vi "Destroy.vi"(0 "reference in":refnum<class "DP_WebView.lvclass">, 2 "BlankBrowser(True)":bool=TRUE, 5 "Error In":errorcluster) -> (14 "reference out":refnum<class "DP_WebView.lvclass">, 19 "Error Out":errorcluster)   [LabVIEW 2020, in "DP_WebView.lvclass"]
uses:
  DP_WebView.lvclass
  C:/Projects/DependencyViewer/DependencyViewer/DP_WebView_class/data/Microsoft.Web.WebView2.Core.dll
  data/Microsoft.Web.WebView2.Core.dll
  C:/Projects/DependencyViewer/DependencyViewer/DP_WebView_class/data/Microsoft.Web.WebView2.WinForms.dll
  data/Microsoft.Web.WebView2.WinForms.dll
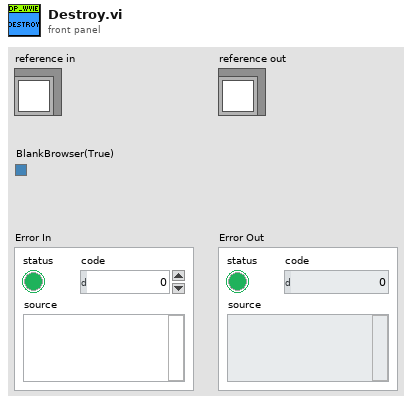
[diagram p1: front panel]
types:
  T1 = typedef "DP_WebView.lvclass/ObjectAttributes.ctl" = cluster{"WebView Container":refnum<k24>, "CoreWebViewRef":refnum<k24>, "Status":i32, "Status Message":string, "User Data Folder":path, "BrowserProcessId":u32}
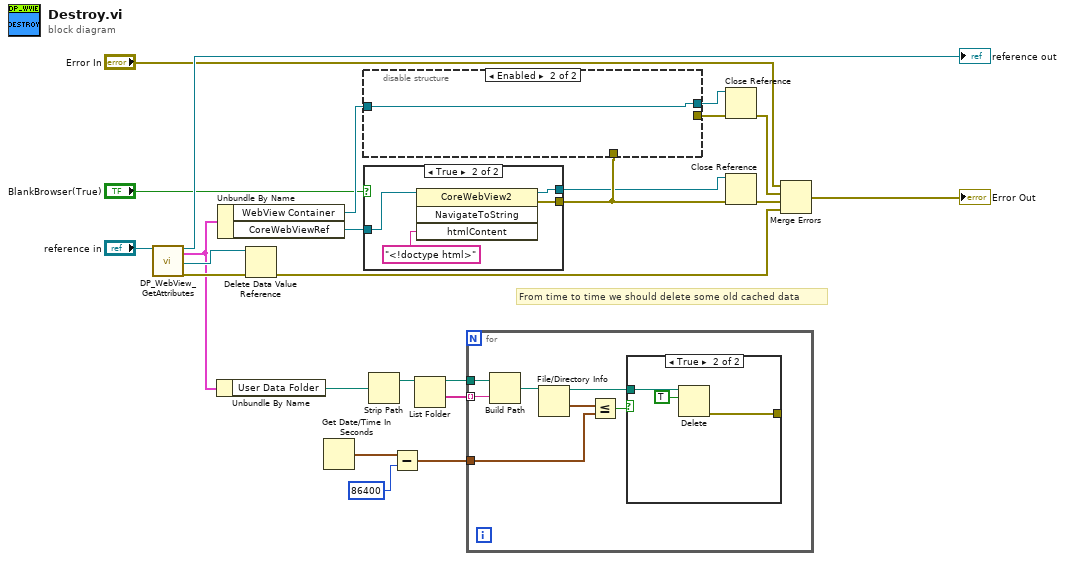
[diagram p0: block diagram]
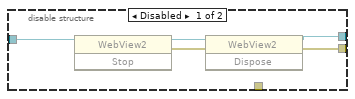
[diagram p4: hidden frame]
diagram:
  # "From time to time we should delete some old cached data"
  n1 = call "DP_WebView_GetAttributes.vi"("reference in"="reference in") -> ("reference out"=→"reference out":refnum<class "DP_WebView.lvclass">, "Data"=w10:T1, "DataRef"=w21:refnum<data-value>, "error out"=w22:errorcluster)  [unwired: 15 in]
  n2 = Unbundle By Name(w10) -> ("User Data Folder"=w7:path)
  n3 = Unbundle By Name(w10) -> ("WebView Container"=w19:refnum<k24>, "CoreWebViewRef"=w12:refnum<k24>)
  n4 = Delete Data Value Reference(data value reference=w21, error in=w22) -> (error out=w15:errorcluster)  [unwired: 1 out]
  n5 = Get Date/Time In Seconds() -> (seconds since 1Jan1904=w3:timestamp)
  n6 = case shown="True" "BlankBrowser(True)" {
    tunnel: w12 -> [w25 w29]
    tunnel: [w25 w28] -> w8
    tunnel: [_ w27] -> w9
    frame False {
    }
    frame True {
      n7 = invoke class="CoreWebView2" method="NavigateToString"(reference=w29, "htmlContent"="<!doctype html>") -> (reference out=w28:refnum<k24>, error out=w27:errorcluster)  [unwired: 2 in, 2 out]
    }
  }
  n8 = disable-structure shown="Enabled" {
    disable-tunnel: [w30 _] -> w14
    disable-tunnel: [w31 w35] -> w13
    disable-tunnel: w19 -> [w34 w35]
    disable-tunnel: w9 -> [_ _]
    frame Disabled {
      n9 = invoke class="WebView2" method="Stop"(reference=w34) -> (reference out=w33:refnum<k24>, error out=w32:errorcluster)  [unwired: 2 in, 1 out]
      n10 = invoke class="WebView2" method="Dispose"(reference=w33, error in=w32) -> (reference out=w31:refnum<k24>, error out=w30:errorcluster)  [unwired: 1 in, 1 out]
    }
    frame Enabled {
    }
  }
  n11 = Strip Path(path=w7) -> (stripped path=w6:path)  [unwired: 1 out]
  n12 = Subtract(x=w3, y=86400) -> (x-y=w1:timestamp)
  n13 = List Folder(path=w6) -> (path out=w4:path, folder names=w5:string[])  [unwired: 3 in, 2 out]
  n14 = for {
    tunnel: w5 -> [w41] mode=indexing
    tunnel: w4 -> [w42]
    tunnel: w1 -> [w38]
    n15 = Build Path(base path=w42, name or relative path=w41) -> (appended path=w40:path)
    n16 = File/Directory Info(path=w40) -> (path out=w36:path, last mod=w39:timestamp)  [unwired: 1 in, 5 out]
    n17 = Less Or Equal?(x=w39, y=w38) -> (x <= y?=w37:bool)
    n18 = case shown="True" w37 {
      tunnel: w36 -> [_ w45]
      tunnel: [_ w43] -> _
      frame False {
      }
      frame True {
        n19 = Delete(path (use dialog)=w45, entire hierarchy (F)=TRUE) -> (error out=w43:errorcluster)  [unwired: 3 in, 2 out]
      }
    }
  }
  n20 = Close Reference(reference=w13, error in (no error)=w14) -> (error out=w20:errorcluster)
  n21 = Close Reference(reference=w8, error in (no error)=w9) -> (error out=w18:errorcluster)
  n22 = Merge Errors("Error In", w20, w18, w15) -> (→"Error Out":errorcluster)
